vi "Bezier Curve.vi"(9 "position":dbl[](array[numeric]), 10 "percision":dbl, 11 "ctrl points":cluster{dbl, dbl}[](array[cluster])) -> (3 "curve":T1)   [LabVIEW 2019]
uses:
  Types/Bezier Curve.ctl
  <vilib>/Analysis/2dsp.llb/2D Inverse Complex FFT.vi
  <vilib>/Analysis/NI_AALPro.lvlib
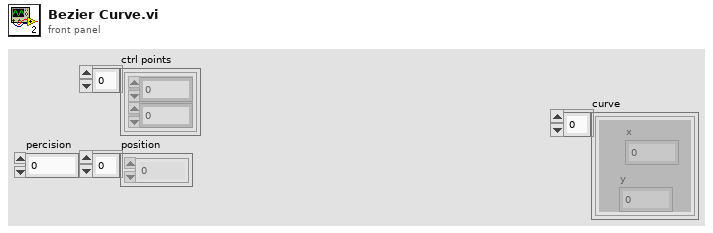
[diagram p1: front panel]
types:
  T1 = typedef "Bezier Curve.ctl" = cluster{"x":dbl, "y":dbl}[]
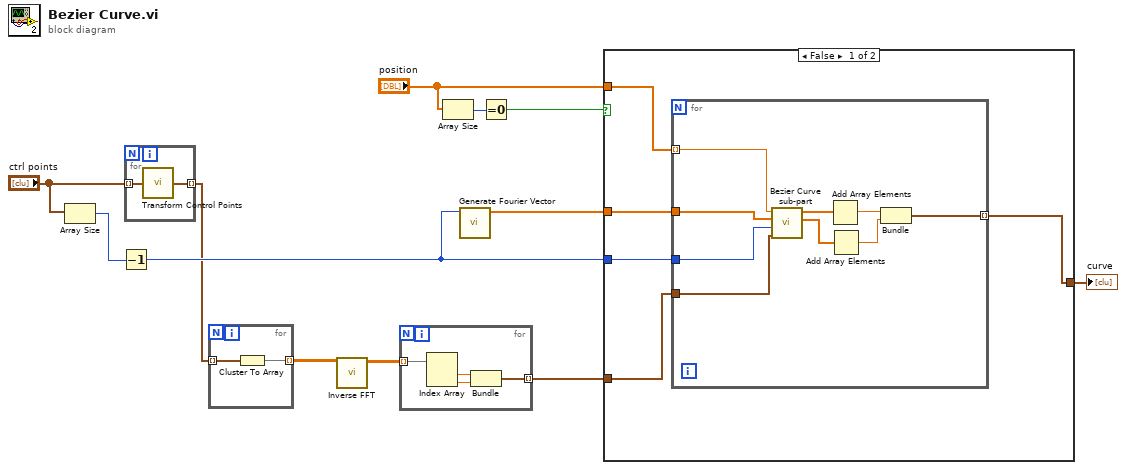
[diagram p0: block diagram]
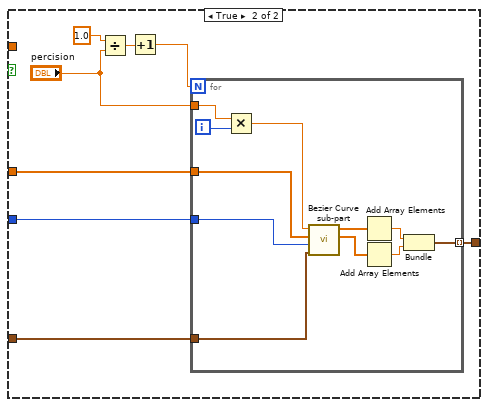
[diagram p2: hidden frame]
diagram:
  n1 = Array Size(array="ctrl points") -> (size(s)=w6:i32)
  n2 = Decrement(x=w6) -> (x-1=w5:i32)
  n3 = for {
    tunnel: "ctrl points" -> [w14] mode=indexing
    tunnel: [w13] -> w4 mode=indexing
    n4 = call "Transform Control Points.vi"("ctrl pt"=w14) -> ("ctrl pt out"=w13:cluster{dbl, dbl})
  }
  n5 = for {
    tunnel: w4 -> [w16] mode=indexing
    tunnel: [w15] -> w12 mode=indexing
    n6 = Cluster To Array(cluster=w16) -> (array=w15:dbl[])
  }
  n7 = call-poly <vilib>:"Inverse FFT.vi"("FFT {x}"=w12) -> ("X"=w11:cdb[][])  [unwired: 9 in, 1 out]
  n8 = for {
    tunnel: w11 -> [w20] mode=indexing
    tunnel: [w17] -> w10 mode=indexing
    n9 = Index Array(array=w20) -> (element #1=w19:cdb, element #2=w18:cdb)  [unwired: 2 in]
    n10 = Bundle(w19, w18) -> (w17:cluster{cdb, cdb})  [unwired: 1 in]
  }
  n11 = Array Size(array="position") -> (size(s)=w3:i32)
  n12 = call "Generate Fourier Vector.vi"("degree"=w5) -> ("Fourier Matrix"=w8:cdb[])  [unwired: 10 in]
  n13 = Equal To 0?(x=w3) -> (x = 0?=w2:bool)
  n14 = case shown="False" w2 {
    tunnel: w10 -> [w22 w41]
    tunnel: [w21 w40] -> w9
    tunnel: w8 -> [w24 w39]
    tunnel: w5 -> [w23 w36]
    tunnel: "position" -> [w25 _]
    frame False {
      n15 = for {
        tunnel: w25 -> [w34] mode=indexing
        tunnel: w24 -> [w33]
        tunnel: w23 -> [w32]
        tunnel: w22 -> [w31]
        tunnel: [w26] -> w21 mode=indexing
        n16 = call "Bezier Curve sub-part.vi"("Q"=w31, "degree"=w32, "Fourier Matrix"=w33, "position"=w34) -> ("y arr"=w29:dbl[], "x arr"=w30:dbl[])  [unwired: 6 in]
        n17 = Add Array Elements(numeric array=w30) -> (sum=w28:dbl)
        n18 = Add Array Elements(numeric array=w29) -> (sum=w27:dbl)
        n19 = Bundle(w28, w27) -> (w26:cluster{dbl, dbl})  [unwired: 1 in]
      }
    }
    frame True {
      n20 = Divide(x=1.0, y="percision") -> (x/y=w38:dbl)
      n21 = Increment(x=w38) -> (x+1=w37:dbl)
      n22 = for {
        N: w37 -> [_]
        tunnel: "percision" -> [w46]
        tunnel: w36 -> [w44]
        tunnel: w41 -> [w43]
        tunnel: [w47] -> w40 mode=indexing
        tunnel: w39 -> [w45]
        i -> [w53]
        n23 = Multiply(x=w46, y=w53) -> (x*y=w52:dbl)
        n24 = call "Bezier Curve sub-part.vi"("Q"=w43, "degree"=w44, "Fourier Matrix"=w45, "position"=w52) -> ("y arr"=w50:dbl[], "x arr"=w51:dbl[])  [unwired: 6 in]
        n25 = Add Array Elements(numeric array=w51) -> (sum=w48:dbl)
        n26 = Add Array Elements(numeric array=w50) -> (sum=w49:dbl)
        n27 = Bundle(w48, w49) -> (w47:cluster{dbl, dbl})  [unwired: 1 in]
      }
    }
  }
  "curve" <- w9
